vi "Do.vi"(8 "error in (no error)":errorcluster, 10 "Actor in":refnum<class "Actor.lvclass">, 11 "stream_TTTR Msg":refnum<class "stream_TTTR Msg.lvclass">) -> (0 "error out":errorcluster, 2 "Actor out":refnum<class "Actor.lvclass">)   [LabVIEW 2015, in "stream_TTTR Msg.lvclass"]
doc: "This VI delivers the message to the actor by calling the appropriate method(s) on the actor."
uses:
  stream_TTTR Msg.lvclass
  <vilib>/ActorFramework/Actor/Actor.lvclass
  hydraharp_panel/hydraharp_panel.lvclass
  stream_TTTR Msg.lvclass/stream_TTTR Msg.ctl
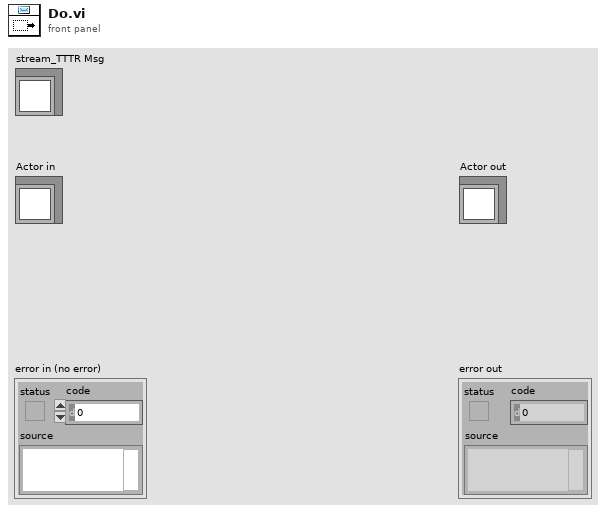
[diagram p1: front panel]
types:
  T1 = typedef "hydraharp_action_on_records.ctl" = enum16{"stream_to_file", "correlate", "stream to file and correlate"}
  T2 = typedef "hpanel_correlation_settings.ctl" = cluster{"Lag Settings":T3, "Ch1":u8, "Ch2":u8}
  T3 = typedef "hydraharp_correlation_lag_settings.ctl" = cluster{"time_start":T4, "time_end":T4, "coarseness":i64}
  T4 = typedef "hydraharp_time_decades.ctl" = i64
  T5 = typedef "record_type.ctl" = enum16{"Raw Stream", "Processed Records (hdf5)"}
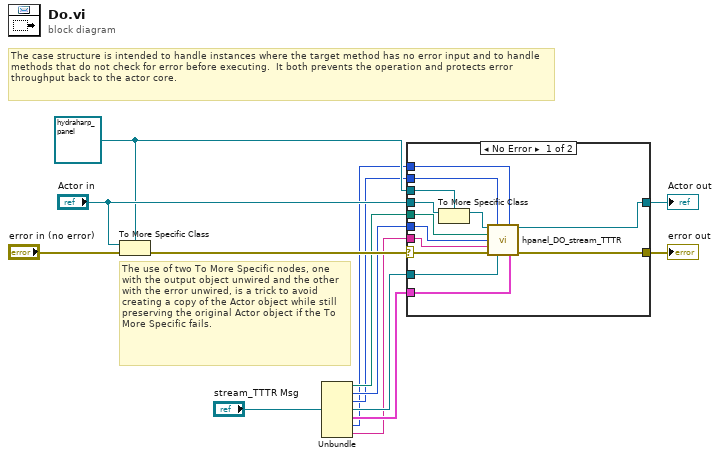
[diagram p0: block diagram]
diagram:
  w8 = refnum<class "hydraharp_panel.lvclass"> refnum ("Actor in")
  # "The use of two To More Specific nodes, one with the output object unwired and the other with the error unwired, is a trick to avoid creating a copy of the Actor object while still preserving the original Actor object if the To More Specific fails."
  # "The case structure is intended to handle instances where the target method has no error input and to handle methods that do not check for error before executing.  It both prevents the operation and protects error throughput back to the actor core."
  n1 = To More Specific Class(target class=w8, reference="Actor in", error in="error in (no error)") -> (error out=w12:errorcluster)  [unwired: 1 out]
  n2 = Unbundle("stream_TTTR Msg") -> (w7:path, w6:T1, w5:i32, w4:refnum<event-registration>, w3:T2, w2:T5, w1:string)
  n3 = case shown="No Error" w12 {
    selector: w12 -> [w25 w29]
    tunnel: [w27 w29] -> w11
    tunnel: [w26 w28] -> w10
    tunnel: "Actor in" -> [w24 w28]
    tunnel: w8 -> [w23 _]
    tunnel: w7 -> [w21 _]
    tunnel: w6 -> [w20 _]
    tunnel: w5 -> [w19 _]
    tunnel: w4 -> [w17 _]
    tunnel: w3 -> [w16 _]
    tunnel: w2 -> [w18 _]
    tunnel: w1 -> [w15 _]
    frame No Error {
      n4 = To More Specific Class(target class=w23, reference=w24) -> (specific class reference=w22:refnum<class "hydraharp_panel.lvclass">)  [unwired: 1 in, 1 out]
      n5 = call "hpanel_DO_stream_TTTR.vi"("hydraharp_panel in"=w22, "acq_time"=w19, "Record Type"=w18, "fifo_stream_path"=w21, "action_for_records"=w20, "Stream Notes"=w15, "error in (no error)"=w25, "stop_fifo_event"=w17, "Correlation_settings"=w16) -> ("hydraharp_panel out"=w26:refnum<class "hydraharp_panel.lvclass">, "error out"=w27:errorcluster)  [unwired: 5 in]
    }
    frame Error {
      # "If type check fails, pass the original object out again."
    }
  }
  "error out" <- w11
  "Actor out" <- w10
